vi "Initialise GMap.vi"(8 "error in (no error)":errorcluster, 10 "Mini Map":refnum<k24>(container), 11 "Main Map":refnum<k24>(container)) -> (0 "Error Out":errorcluster)   [LabVIEW 2014]
uses:
  C:/Robotic Systems/Products/AgFalcon/Software/Ground Station/Data/Mapping DLL/GMap.NET.WindowsForms.dll
  Data/Mapping DLL/GMap.NET.WindowsForms.dll
  Reference/Controls/Mapping References.ctl
  C:/Robotic Systems/Products/AgFalcon/Software/Ground Station/Data/Mapping DLL/GMap.NET.Core.dll
  Data/Mapping DLL/GMap.NET.Core.dll
  Settings File/SubVI/Load Last Home Lat.vi
  Settings File/SubVI/Load Last Home Lon.vi
panel:
  in  "error in (no error) 2":errorcluster
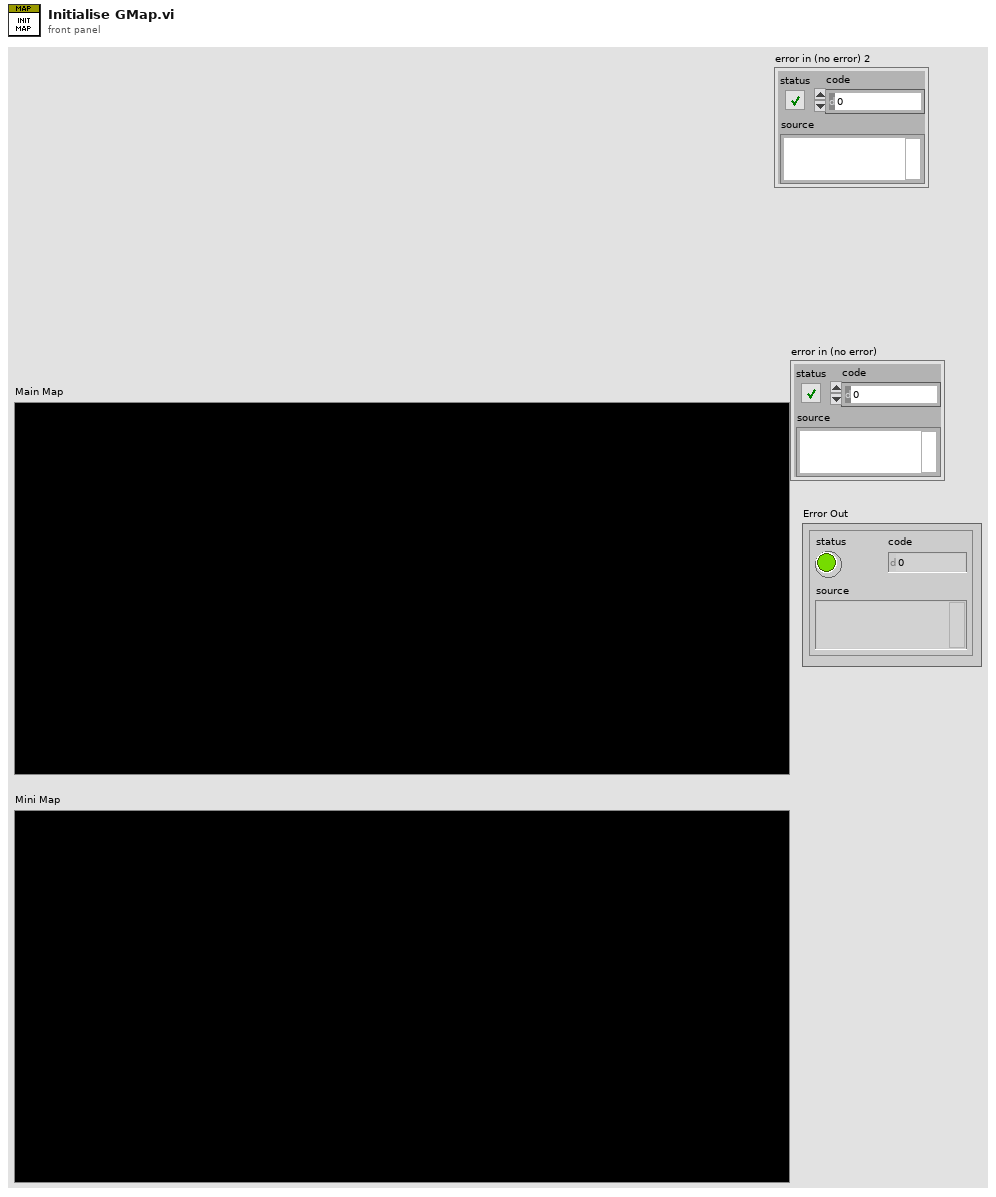
[diagram p1: front panel]
types:
  T1 = typedef "Mapping References.ctl" = cluster{"Main Map DLL Reference":refnum<k24>, "Main Map Control Reference":refnum<k24>, "Mini Map DLL Reference":refnum<k24>, "Mini Map Control Reference":refnum<k24>}
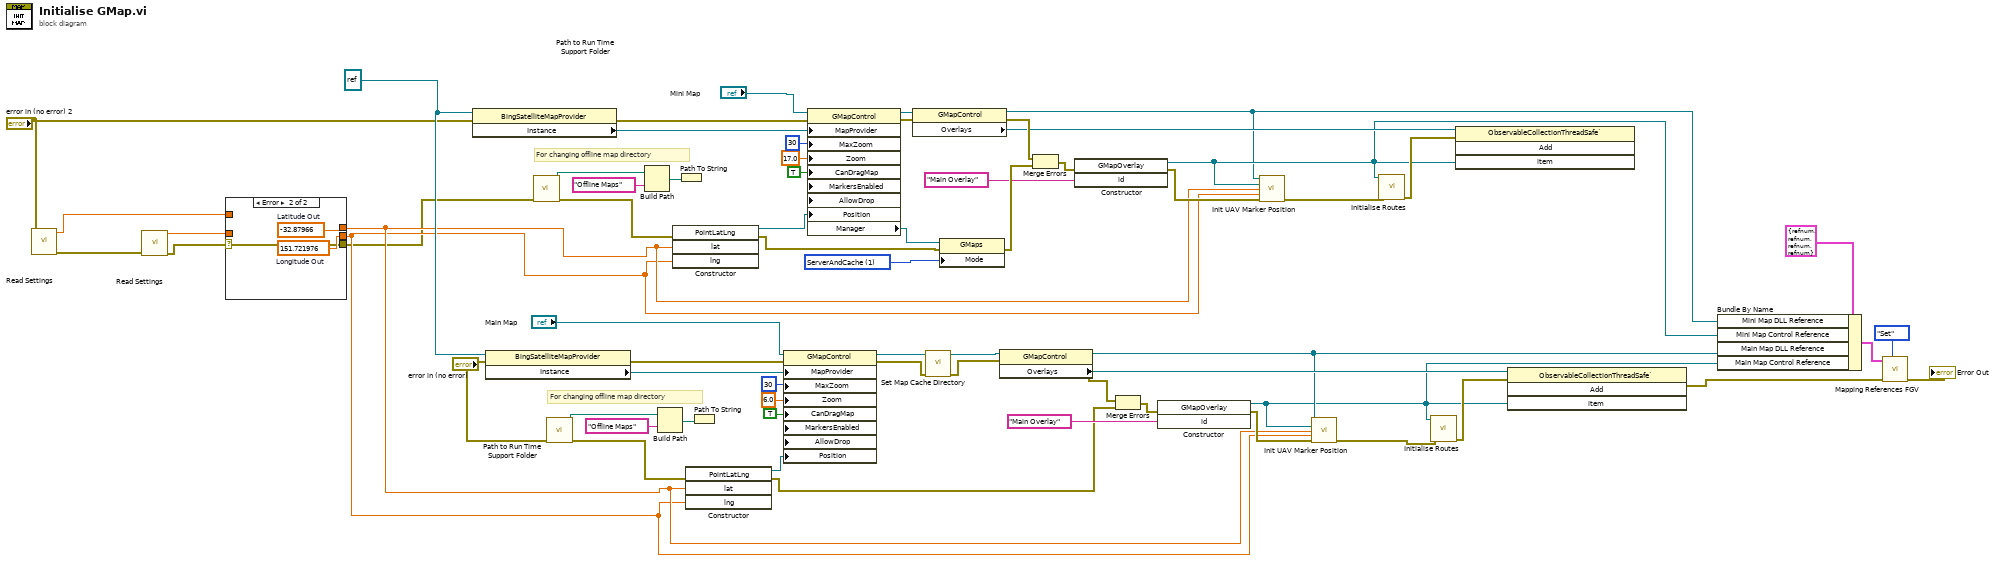
[diagram p0: block diagram]
diagram:
  w31 = 1 items=["ServerOnly", "ServerAndCache", "CacheOnly"] ("Mode")
  w26 = TRUE ("CanDragMap")
  w18 = refnum<k24> refnum (".NET Container Reference")
  w63 = TRUE ("CanDragMap")
  # "For changing offline map directory"
  # "For changing offline map directory"
  n1 = call-poly "Read Settings.vi"("Error In"="error in (no error) 2") -> ("error out"=w12:errorcluster, "Home Lat"=w10:dbl)  [unwired: 9 in]
  n2 = call-poly "Read Settings.vi"("Error In"=w12) -> ("error out"=w11:errorcluster, "Home Lon"=w9:dbl)  [unwired: 9 in]
  n3 = case shown="Error" w11 {
    selector: w11 -> [w67 w70]
    tunnel: w10 -> [w69 _]
    tunnel: w9 -> [w68 _]
    tunnel: [w69 w72] -> w8
    tunnel: [w68 w71] -> w7
    tunnel: [w67 w70] -> w6
    frame No Error {
    }
    frame Error {
      w71 = 151.721976  # Longitude Out
      w72 = -32.87966  # Latitude Out
    }
  }
  n4 = property class="BingSatelliteMapProvider"(reference=w18, error in="error in (no error) 2") -> (error out=w22:errorcluster, "Instance"=w23:refnum<k24>)  [unwired: 1 out]
  n5 = property class="BingSatelliteMapProvider"(reference=w18, error in="error in (no error)") -> (error out=w15:errorcluster, "Instance"=w66:refnum<k24>)  [unwired: 1 out]
  n6 = call "Path to Run Time Support Folder.vi"("Error In"=w6) -> ("Error Out"=w43:errorcluster, "Path To Run Time Support Folder"=w42:path)  [unwired: 9 in]
  n7 = call "Path to Run Time Support Folder.vi"("Error In"="error in (no error)") -> ("Error Out"=w49:errorcluster, "Path To Run Time Support Folder"=w51:path)  [unwired: 9 in]
  n8 = Build Path(base path=w42, name or relative path="Offline Maps") -> (appended path=w41:path)
  n9 = Build Path(base path=w51, name or relative path="Offline Maps") -> (appended path=w52:path)
  n10 = constructor class="PointLatLng"(error in=w43, "lat"=w8, "lng"=w7) -> (reference out=w29:refnum<k24>, error out=w32:errorcluster)  [unwired: 2 in, 3 out]
  n11 = Path To String(path=w41) -> ()  [unwired: 1 out]
  n12 = constructor class="PointLatLng"(error in=w49, "lat"=w8, "lng"=w7) -> (reference out=w61:refnum<k24>, error out=w1:errorcluster)  [unwired: 2 in, 3 out]
  n13 = Path To String(path=w52) -> ()  [unwired: 1 out]
  n14 = property class="GMapControl"(reference="Main Map", error in=w15, "MapProvider"=w66, "MaxZoom"=30, "Zoom"=6.0, "CanDragMap"=w63, "MarkersEnabled"=w63, "AllowDrop"=w63, "Position"=w61) -> (reference out=w4:refnum<k24>, error out=w3:errorcluster)
  n15 = property class="GMapControl"(reference="Mini Map", error in=w22, "MapProvider"=w23, "MaxZoom"=30, "Zoom"=17.0, "CanDragMap"=w26, "MarkersEnabled"=w26, "AllowDrop"=w26, "Position"=w29) -> (reference out=w34:refnum<k24>, error out=w27:errorcluster, "Manager"=w30:refnum<k24>)
  n16 = property class="GMapControl"(reference=w34, error in=w27) -> (reference out=w19:refnum<k24>, error out=w39:errorcluster, "Overlays"=w33:refnum<k24>)
  n17 = call "Set Map Cache Directory.vi"("Error In"=w3, "Map Ref"=w4) -> ("Error Out"=w2:errorcluster, "Map Ref 2"=w5:refnum<k24>)  [unwired: 8 in]
  n18 = property class="GMaps"(reference=w30, error in=w32, "Mode"=w31) -> (error out=w40:errorcluster)  [unwired: 1 out]
  n19 = property class="GMapControl"(reference=w5, error in=w2) -> (reference out=w56:refnum<k24>, error out=w53:errorcluster, "Overlays"=w60:refnum<k24>)
  n20 = Merge Errors(w39, w40) -> (w38:errorcluster)
  n21 = constructor class="GMapOverlay"(error in=w38, "id"="Main Overlay") -> (reference out=w20:refnum<k24>, error out=w35:errorcluster)  [unwired: 2 in, 2 out]
  n22 = Merge Errors(w53, w1) -> (w54:errorcluster)
  n23 = constructor class="GMapOverlay"(error in=w54, "id"="Main Overlay") -> (reference out=w55:refnum<k24>, error out=w59:errorcluster)  [unwired: 2 in, 2 out]
  n24 = call "Init UAV Marker Position.vi"("GMAP Control ref"=w19, "Overlay Ref"=w20, "lat"=w8, "lng"=w7, "error in (no error)"=w35) -> ("error out"=w36:errorcluster)  [unwired: 10 in]
  n25 = call "Init UAV Marker Position.vi"("GMAP Control ref"=w56, "Overlay Ref"=w55, "lat"=w8, "lng"=w7, "error in (no error)"=w59) -> ("error out"=w14:errorcluster)  [unwired: 10 in]
  n26 = call "Initialise Routes.vi"("error in (no error)"=w36, "Main Overlay"=w20) -> ("error out"=w37:errorcluster)  [unwired: 9 in]
  n27 = call "Initialise Routes.vi"("error in (no error)"=w14, "Main Overlay"=w55) -> ("error out"=w58:errorcluster)  [unwired: 9 in]
  n28 = invoke class="ObservableCollectionThreadSafe`" method="Add"(reference=w33, error in=w37, "item"=w20) -> ()  [unwired: 1 in, 4 out]
  n29 = invoke class="ObservableCollectionThreadSafe`" method="Add"(reference=w60, error in=w58, "item"=w55) -> (error out=w17:errorcluster)  [unwired: 1 in, 3 out]
  n30 = Bundle By Name(cluster=T1 {"Main Map DLL Reference"=refnum, "Main Map Control Reference"=refnum, "Mini Map DLL Reference"=refnum, "Mini Map Control Reference"=refnum} ("Map References"), "Mini Map DLL Reference"=w19, "Mini Map Control Reference"=w20, "Main Map DLL Reference"=w56, "Main Map Control Reference"=w55) -> (w47:T1)
  n31 = call "Mapping References FGV.vi"("Method"=enum16{"Get", "Set"}."Set", "Error In"=w17, "Map References"=w47) -> ("Error Out"=→"Error Out":errorcluster)  [unwired: 7 in, 1 out]
